vi "Pulse Güncel Deneme.vi"() -> ()   [LabVIEW 2019]
uses:
  <vilib>/Utility/error.llb/DialogType.ctl
  <vilib>/DAQmx/create/channels.llb/DAQmx Create Channel (CO-Pulse Generation-Time).vi
  <vilib>/DAQmx/configure/timing.llb/DAQmx Timing (Implicit).vi
  <resource>/objmgr/daqmx.rc
  <vilib>/DAQmx/create/channels.llb/DAQmx Create Channel (CI-Count Edges).vi
  <vilib>/DAQmx/configure/timing.llb/DAQmx Timing (Sample Clock).vi
  <vilib>/DAQmx/read.llb/DAQmx Read (Counter 1D U32 1Chan NSamp).vi
panel:
  in  "Trigger Type":T1(tab)
  in  "Edge":i32(ring)=10280 items=["Rising"=10280, "Falling"=10171]
  in  "Digital Trigger Source":tag
  in  "Pause When":i32(ring)=10192 items=["High"=10192, "Low"=10214]
  in  "Pause Trigger Source":tag
  in  "Count Reset Terminal":tag
  in  "Edge 2":i32(ring)=10280 items=["Rising"=10280, "Falling"=10171]
  in  "Sample Rate":dbl=1000.0
  in  "Sample Clock Source":tag="PFI0"
  in  "Samples per Loop":i32=100
  in  "Stop 2":bool
  out "Data":u32[](array[numeric])
  in  "Stop":bool
  # "To configure and use a trigger or the count reset you must have the necessary tab selected above.  Not all hardware supports the above options--refer to your device documentation for more info."
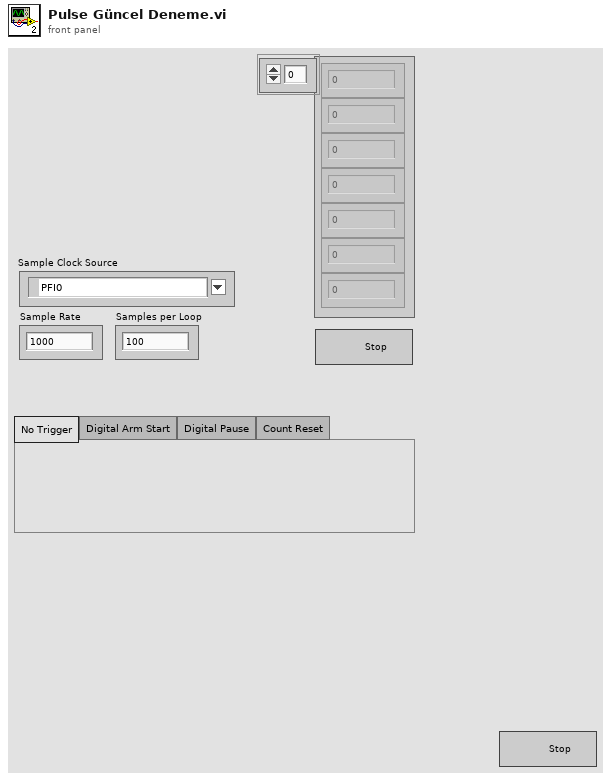
[diagram p1: front panel]
types:
  T1 = enum32{"No Trigger", "Digital Arm Start", "Digital Pause", "Count Reset"}
  T2 = typedef "DialogType.ctl" = u16
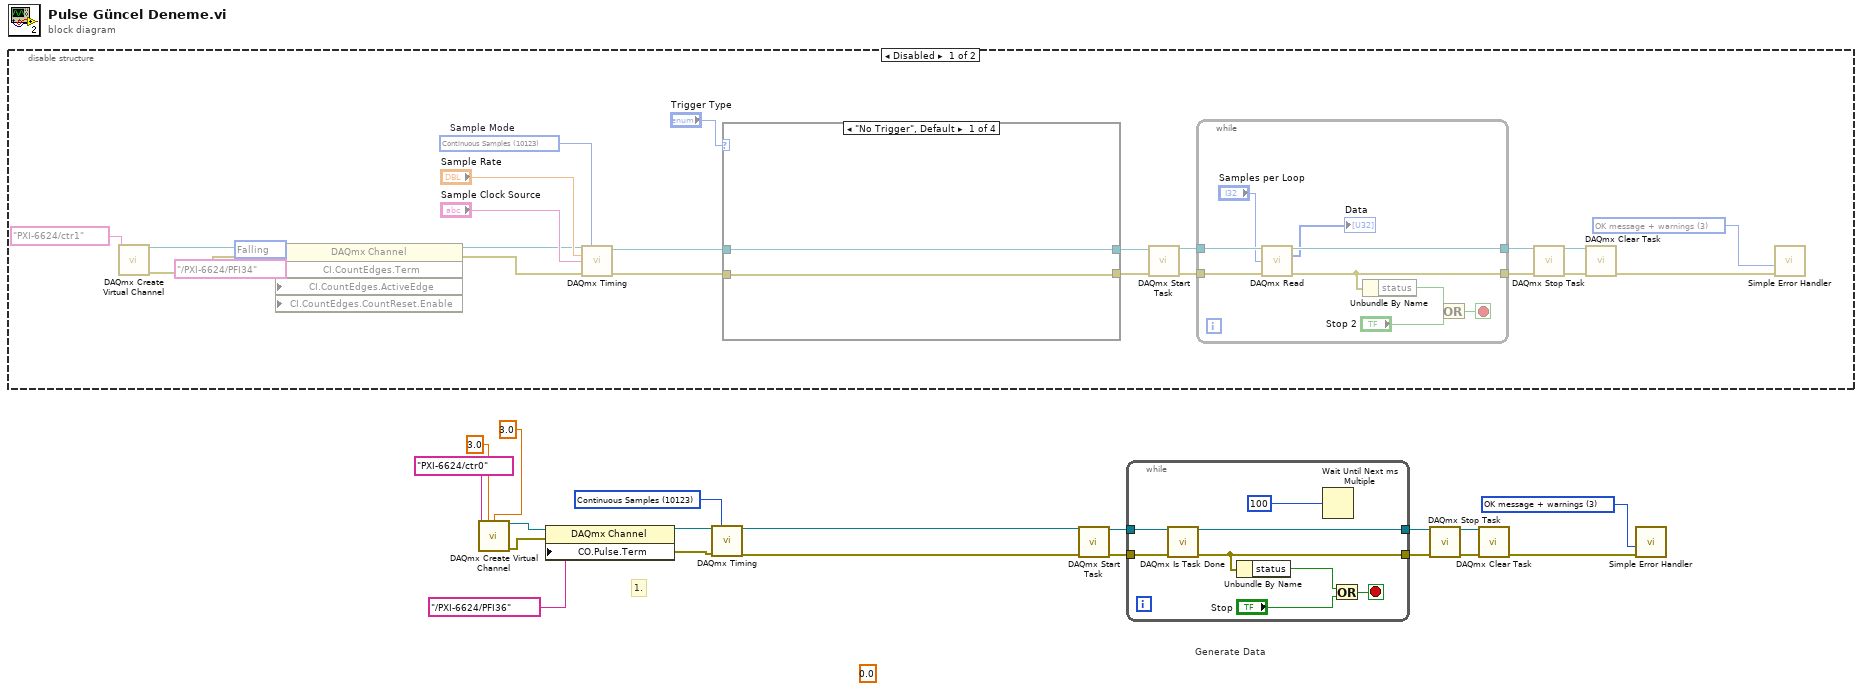
[diagram p0: block diagram]
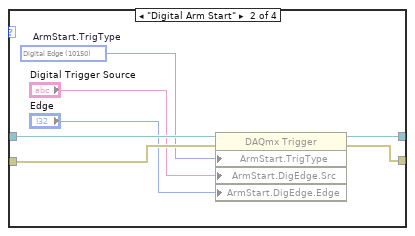
[diagram p2: hidden frame]
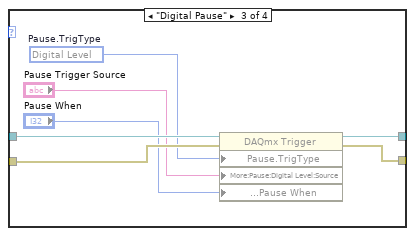
[diagram p3: hidden frame]
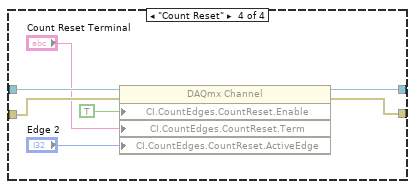
[diagram p4: hidden frame]
diagram:
  (unwired) 0.0 ("AIConv.DigFltr.MinPulseWidth")
  w9 = 10123 items=["Finite Samples"=10178, "Continuous Samples"=10123, "Hardware Timed Single Point"=12522] ("sample mode")
  w12 = T2 3 items=["no dialog", "OK message", "continue or stop message", "OK message + warnings", "continue/stop + warnings"] ("type of dialog (OK msg:1)")
  # "1."
  # "Generate Data"
  n1 = disable-structure shown="Disabled" {
    frame Disabled {
      w20 = 10171 items=["Rising"=10280, "Falling"=10171] ("CI.CountEdges.ActiveEdge")
      w23 = T2 3 items=["no dialog", "OK message", "continue or stop message", "OK message + warnings", "continue/stop + warnings"] ("type of dialog (OK msg:1)")
      w42 = 10123 items=["Finite Samples"=10178, "Continuous Samples"=10123, "Hardware Timed Single Point"=12522]  # Sample Mode
      n2 = call-poly <vilib>:"DAQmx Create Virtual Channel.vi"("counter"=tag "PXI-6624/ctr1") -> ("task out"=w36:refnum<k21>, "error out"=w33:errorcluster)  [unwired: 13 in]
      n3 = property class="DAQmx Channel" props=["CI.CountEdges.Term", "CI.CountEdges.ActiveEdge", "CI.CountEdges.CountReset.Enable"](reference=w36, error in=w33, "CI.CountEdges.Term"=tag "/PXI-6624/PFI34", "CI.CountEdges.ActiveEdge"=w20) -> (reference out=w35:refnum<k21>, error out=w34:errorcluster)  [unwired: 1 in]
      n4 = call-poly <vilib>:"DAQmx Timing.vi"("task/channels in"=w35, "sample mode"=w42, "rate"="Sample Rate", "source"="Sample Clock Source", "error in"=w34) -> ("task out"=w29:refnum<k21>, "error out"=w28:errorcluster)  [unwired: 9 in]
      n5 = case shown="\"No Trigger\", Default" "Trigger Type" {
        tunnel: w29 -> [w44 w51 w58 w65]
        tunnel: w28 -> [w43 w48 w55 w62]
        tunnel: [w44 w50 w57 w64] -> w30
        tunnel: [w43 w49 w56 w63] -> w31
        frame "No Trigger", Default {
        }
        frame "Digital Arm Start" {
          w45 = 10150 items=["Digital Edge"=10150, "None"=10230]  # ArmStart.TrigType
          n6 = property class="DAQmx Trigger"(reference=w51, error in=w48, "ArmStart.TrigType"=w45, "ArmStart.DigEdge.Src"="Digital Trigger Source", "ArmStart.DigEdge.Edge"="Edge") -> (reference out=w50:refnum<k21>, error out=w49:errorcluster)
        }
        frame "Digital Pause" {
          w54 = 10152 items=["Analog Level"=10101, "Analog Window"=10103, "Digital Level"=10152, "Digital Pattern"=10398, "None"=10230]  # Pause.TrigType
          n7 = property class="DAQmx Trigger"(reference=w58, error in=w55, "Pause.TrigType"=w54, "More:Pause:Digital Level:Source"="Pause Trigger Source", "More:Pause:Digital Level:Pause When"="Pause When") -> (reference out=w57:refnum<k21>, error out=w56:errorcluster)
        }
        frame "Count Reset" {
          n8 = property class="DAQmx Channel"(reference=w65, error in=w62, "CI.CountEdges.CountReset.Enable"=TRUE, "CI.CountEdges.CountReset.Term"="Count Reset Terminal", "CI.CountEdges.CountReset.ActiveEdge"="Edge 2") -> (reference out=w64:refnum<k21>, error out=w63:errorcluster)
        }
      }
      n9 = call <vilib>:"DAQmx Start Task.vi"("task/channels in"=w30, "error in"=w31) -> ("task out"=w41:refnum<k21>, "error out"=w40:errorcluster)  [unwired: 12 in]
      n10 = while {
        tunnel: w41 -> [w74]
        tunnel: w40 -> [w73]
        tunnel: [w70] -> w26
        tunnel: [w71] -> w27
        stop <- w72 stop-if-true
        n11 = call-poly <vilib>:"DAQmx Read.vi"("task/channels in"=w74, "number of samples per channel"="Samples per Loop", "error in"=w73) -> ("task out"=w71:refnum<k21>, "data"=→"Data":u32[], "error out"=w70:errorcluster)  [unwired: 10 in]
        n12 = Unbundle By Name(w70) -> ("status"=w69:bool)
        n13 = Or(x=w69, y="Stop 2") -> (x .or. y?=w72:bool)
      }
      n14 = call <vilib>:"DAQmx Stop Task.vi"("task/channels in"=w27, "error in"=w26) -> ("task out"=w24:refnum<k21>, "error out"=w25:errorcluster)  [unwired: 12 in]
      n15 = call <vilib>:"DAQmx Clear Task.vi"("task in"=w24, "error in"=w25) -> ("error out"=w39:errorcluster)  [unwired: 13 in]
      n16 = call <vilib>:"Simple Error Handler.vi"("type of dialog (OK msg:1)"=w23, "error in (no error)"=w39) -> ()  [unwired: 3 in, 5 out]
    }
    frame Enabled {
    }
  }
  n17 = call-poly <vilib>:"DAQmx Create Virtual Channel.vi"("high time"=3.0, "low time"=3.0, "counter"=tag "PXI-6624/ctr0") -> ("task out"=w4:refnum<k21>, "error out"=w5:errorcluster)  [unwired: 11 in]
  n18 = property class="DAQmx Channel"(reference=w4, error in=w5, "CO.Pulse.Term"=tag "/PXI-6624/PFI36") -> (reference out=w11:refnum<k21>, error out=w10:errorcluster)
  n19 = call-poly <vilib>:"DAQmx Timing.vi"("task/channels in"=w11, "sample mode"=w9, "error in"=w10) -> ("task out"=w2:refnum<k21>, "error out"=w1:errorcluster)  [unwired: 11 in]
  n20 = call <vilib>:"DAQmx Start Task.vi"("task/channels in"=w2, "error in"=w1) -> ("task out"=w19:refnum<k21>, "error out"=w18:errorcluster)  [unwired: 12 in]
  n21 = while {
    tunnel: w19 -> [w82]
    tunnel: w18 -> [w81]
    tunnel: [w78] -> w13
    tunnel: [w79] -> w14
    stop <- w80 stop-if-true
    n22 = call <vilib>:"DAQmx Is Task Done.vi"("task/channels in"=w82, "error in"=w81) -> ("task out"=w79:refnum<k21>, "error out"=w78:errorcluster)  [unwired: 11 in, 1 out]
    n23 = Unbundle By Name(w78) -> ("status"=w77:bool)
    n24 = Wait Until Next ms Multiple(millisecond multiple=u32 100) -> ()  [unwired: 1 out]
    n25 = Or(x=w77, y="Stop") -> (x .or. y?=w80:bool)
  }
  n26 = call <vilib>:"DAQmx Stop Task.vi"("task/channels in"=w14, "error in"=w13) -> ("task out"=w16:refnum<k21>, "error out"=w15:errorcluster)  [unwired: 12 in]
  n27 = call <vilib>:"DAQmx Clear Task.vi"("task in"=w16, "error in"=w15) -> ("error out"=w17:errorcluster)  [unwired: 13 in]
  n28 = call <vilib>:"Simple Error Handler.vi"("type of dialog (OK msg:1)"=w12, "error in (no error)"=w17) -> ()  [unwired: 3 in, 5 out]
